vi "ADO Connection Close.vi"(8 "error in (no error)":errorcluster, 11 "ADODB._Connection In":refnum<k7>) -> (0 "error out":errorcluster, 3 "ADODB._Connection Out":refnum<k7>)   [LabVIEW 2011]
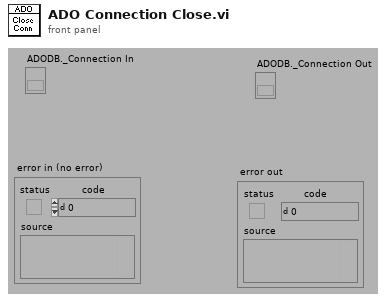
[diagram p1: front panel]
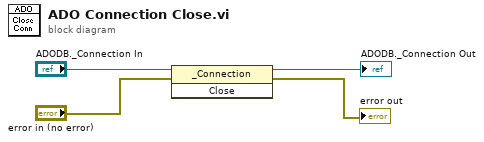
[diagram p0: block diagram]
diagram:
  n1 = invoke class="_Connection" method="Close"(reference="ADODB._Connection In", error in="error in (no error)") -> (reference out=→"ADODB._Connection Out":refnum<k7>, error out=→"error out":errorcluster)  [unwired: 1 in, 1 out]
